vi "sv_Identify Multitone Frequency Pattern.vi"(11 "frequencies":dbl[](array[numeric])) -> (1 "test signal":T1(ring)=enum."test signal not recognized", 2 "valid test signal":bool)   [LabVIEW 2017, in "SoundVib_Distortion.lvlib"]
uses:
  <vilib>/addons/Sound and Vibration/svt_Distortion/SoundVib_Distortion.lvlib
  <vilib>/Analysis/NI_AALPro.lvlib
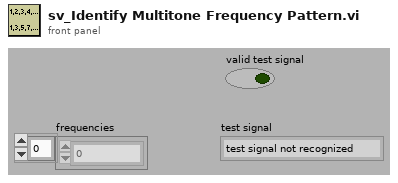
[diagram p1: front panel]
types:
  T1 = enum16{"even-spaced multitone", "square wave", "test signal not recognized"}
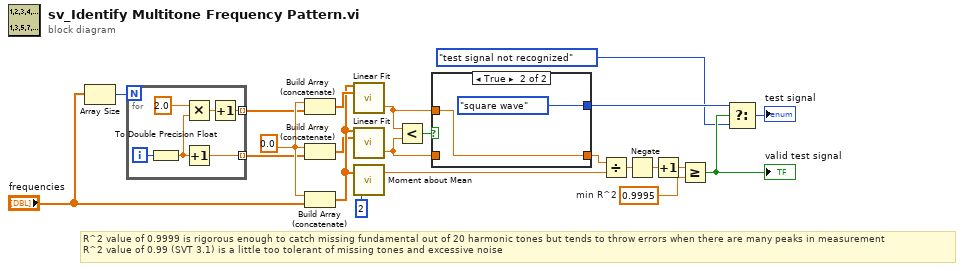
[diagram p0: block diagram]
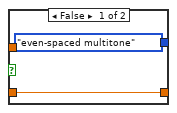
[diagram p2: hidden frame]
diagram:
  w16 = 0.0 ("double precision float")
  w2 = 0.9995  # min R^2
  # "R^2 value of 0.9999 is rigorous enough to catch missing fundamental out of 20 harmonic tones but tends to throw errors when there are many peaks in measurement\nR^2 value of 0.99 (SVT 3.1) is a little too tolerant of missing tones and excessive noise"
  n1 = Array Size(array="frequencies") -> (size(s)=w17:i32)
  n2 = for {
    N: w17 -> [_]
    tunnel: [w25] -> w15 mode=indexing
    tunnel: [w23] -> w14 mode=indexing
    i -> [w28]
    n3 = To Double Precision Float(number=w28) -> (double precision float=w24:dbl)
    n4 = Multiply(x=2.0, y=w24) -> (x*y=w26:dbl)
    n5 = Increment(x=w24) -> (x+1=w23:dbl)
    n6 = Increment(x=w26) -> (x+1=w25:dbl)
  }
  n7 = Build Array (concatenate)(w16, w15) -> (w13:dbl[])
  n8 = Build Array (concatenate)(w16, w14) -> (w11:dbl[])
  n9 = Build Array (concatenate)(w16, "frequencies") -> (w12:dbl[])
  n10 = call <vilib>:"Linear Fit.vi"("Y"=w12, "X"=w13) -> ("residue"=w9:dbl)  [unwired: 9 in, 4 out]
  n11 = call <vilib>:"Linear Fit.vi"("Y"=w12, "X"=w11) -> ("residue"=w8:dbl)  [unwired: 9 in, 4 out]
  n12 = call <vilib>:"Moment about Mean.vi"("order"=2, "X"=w12) -> ("moment"=w20:dbl)  [unwired: 1 out]
  n13 = Less?(x=w9, y=w8) -> (x < y?=w10:bool)
  n14 = case shown="True" w10 {
    tunnel: w9 -> [_ w31]
    tunnel: w8 -> [w30 _]
    tunnel: [T1."even-spaced multitone" T1."square wave"] -> w5
    tunnel: [w30 w31] -> w7
    frame False {
    }
    frame True {
    }
  }
  n15 = Divide(x=w7, y=w20) -> (x/y=w21:dbl)
  n16 = Negate(x=w21) -> (-x=w19:dbl)
  n17 = Increment(x=w19) -> (x+1=w22:dbl)
  n18 = Greater Or Equal?(x=w22, y=w2) -> (x >= y?=w6:bool)
  "valid test signal" <- w6
  n19 = Select(t=w5, s=w6, f=T1."test signal not recognized" ("Enum")) -> (s? t:f=→"test signal":T1)
